vi "Engine.vi"(8 "error in (no error)":errorcluster, 10 "Init if needed (T)":bool=TRUE) -> (0 "error out":errorcluster, 3 "Engine":refnum<class "Engine.lvclass">)   [LabVIEW 2020, in "GLF.lvlib" / "Engine.lvclass"]
uses:
  Engine.lvclass
  Engine.lvclass/Engine.ctl
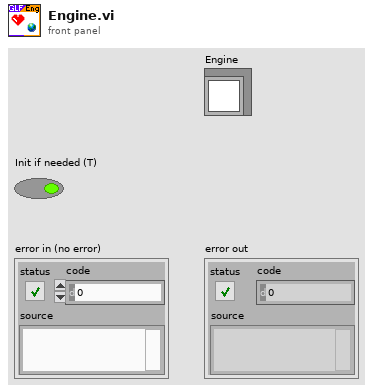
[diagram p1: front panel]
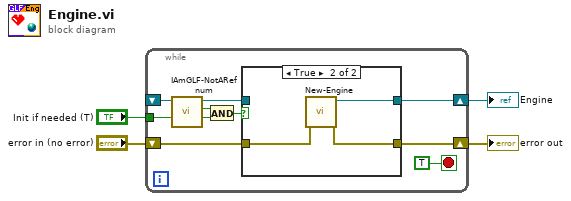
[diagram p0: block diagram]
diagram:
  n1 = while {
    shift-right: [w12] -> w2
    shift-left: _ -> [w9]
    shift-right: [w10] -> w3
    shift-left: "error in (no error)" -> [w11]
    tunnel: "Init if needed (T)" -> [w5]
    stop <- TRUE stop-if-true
    n2 = call-dynamic "IAmGLF-NotARefnum.vi"("Engine in"=w9) -> ("Not A Valid Refnum?"=w7:bool, "Engine out"=w8:refnum<class "Engine.lvclass">)  [unwired: 9 in]
    n3 = And(x=w7, y=w5) -> (x .and. y?=w6:bool)
    n4 = case shown="True" w6 {
      tunnel: [w15 w18] -> w12
      tunnel: w11 -> [w14 w17]
      tunnel: [w14 w16] -> w10
      tunnel: w8 -> [w15 _]
      frame False {
      }
      frame True {
        n5 = call "New-Engine.vi"("error in (no error)"=w17) -> ("error out"=w16:errorcluster, "Engine"=w18:refnum<class "Engine.lvclass">)  [unwired: 9 in]
      }
    }
  }
  "error out" <- w3
  "Engine" <- w2
